vi "Multi-Plex.vi"(6 "Settings":T1, 7 "Prev Outputs":dbl[](array[numeric]), 10 "Inputs":dbl[](array[numeric]), 11 "Control":dbl[](array[numeric])) -> (5 "Outputs":dbl[](array[numeric]))   [LabVIEW 2021, in "Software Multi-Plex Engine.lvlib"]
uses:
  Software Multi-Plex Engine.lvlib
  Shared/Compiled.Settings.ctl
  Shared/Software Multi-Plex Shared.lvlib
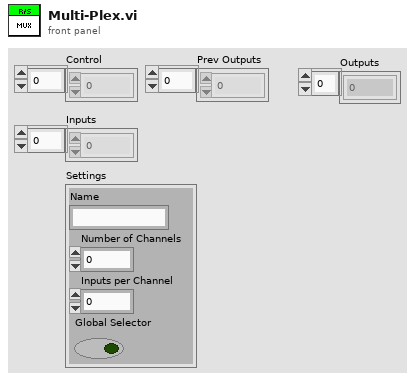
[diagram p1: front panel]
types:
  T1 = typedef "Software Multi-Plex Shared.lvlib/Compiled.Settings.ctl" = cluster{"Name":string, "Number of Channels":i32, "Inputs per Channel":i32, "Global Selector":bool}
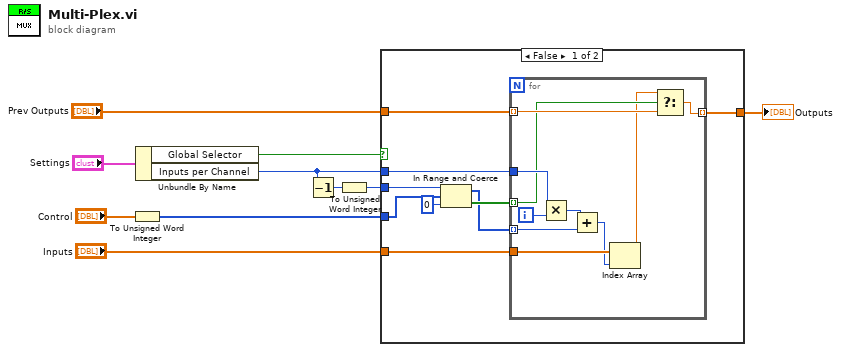
[diagram p0: block diagram]
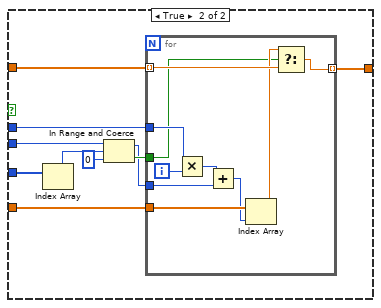
[diagram p2: hidden frame]
diagram:
  n1 = To Unsigned Word Integer(number="Control") -> (unsigned 16bit integer=w4:u16[])
  n2 = Unbundle By Name("Settings") -> ("Global Selector"=w8:bool, "Inputs per Channel"=w3:i32)
  n3 = Decrement(x=w3) -> (x-1=w2:i32)
  n4 = To Unsigned Word Integer(number=w2) -> (unsigned 16bit integer=w1:u16)
  n5 = case shown="False" w8 {
    tunnel: "Inputs" -> [w19 w39]
    tunnel: w3 -> [w17 w38]
    tunnel: [w18 w37] -> w6
    tunnel: "Prev Outputs" -> [w16 w36]
    tunnel: w4 -> [w12 w35]
    tunnel: w1 -> [w15 w33]
    frame False {
      n6 = In Range and Coerce(upper limit=w15, x=w12, lower limit=u16 0) -> (coerced(x)=w11:u16[], In Range?=w13:bool[])
      n7 = for {
        tunnel: w11 -> [w26] mode=indexing
        tunnel: w19 -> [w29]
        tunnel: w17 -> [w28]
        tunnel: [w21] -> w18 mode=indexing
        tunnel: w16 -> [w23] mode=indexing
        tunnel: w13 -> [w22] mode=indexing
        i -> [w27]
        n8 = Multiply(x=w28, y=w27) -> (x*y=w25:i32)
        n9 = Add(x=w25, y=w26) -> (x+y=w24:i32)
        n10 = Index Array(array=w29, index=w24) -> (element=w20:dbl)
        n11 = Select(t=w20, s=w22, f=w23) -> (s? t:f=w21:dbl)
      }
    }
    frame True {
      n12 = Index Array(array=w35) -> (element=w34:u16)  [unwired: 1 in]
      n13 = In Range and Coerce(upper limit=w33, x=w34, lower limit=u16 0) -> (coerced(x)=w30:u16, In Range?=w31:bool)
      n14 = for {
        tunnel: w30 -> [w46]
        tunnel: w39 -> [w49]
        tunnel: w38 -> [w48]
        tunnel: [w41] -> w37 mode=indexing
        tunnel: w36 -> [w43] mode=indexing
        tunnel: w31 -> [w40]
        i -> [w47]
        n15 = Multiply(x=w48, y=w47) -> (x*y=w45:i32)
        n16 = Add(x=w45, y=w46) -> (x+y=w44:i32)
        n17 = Index Array(array=w49, index=w44) -> (element=w42:dbl)
        n18 = Select(t=w42, s=w40, f=w43) -> (s? t:f=w41:dbl)
      }
    }
  }
  "Outputs" <- w6
